vi "SMU.SetVoltage.vi"(8 "error in (no error)":errorcluster, 10 "Voltage, V":dbl, 11 "SMU.Keithley2600 in":refnum<class "SMU.Keithley2600.lvclass">) -> (0 "error out":errorcluster, 3 "SMU.Keithley2600 out":refnum<class "SMU.Keithley2600.lvclass">)   [LabVIEW 2017, in "SMU.Keithley2600.lvclass"]
uses:
  SMU.Keithley2600.lvclass
  <instrlib>/Keithley 2600 Series/Public/Configure/Source/Configure Source (Level).vi
  <instrlib>/Keithley 2600 Series/Keithley 2600 Series.lvlib
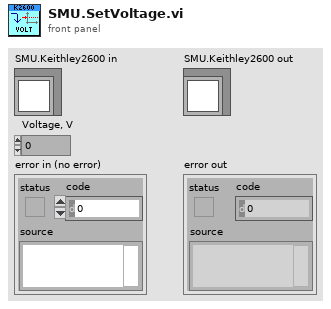
[diagram p1: front panel]
types:
  T1 = typedef "SMU.Keithley2600.lvclass/Resource--Cluster.ctl" = cluster{"VISA resource":refnum<visa-resource-name>, "Channel":i32}
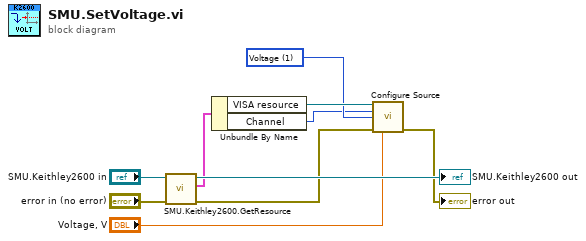
[diagram p0: block diagram]
diagram:
  w5 = 1 items=["Current", "Voltage"] ("Level Type (1: Voltage)")
  n1 = call "SMU.Keithley2600.GetResource.vi"("error in (no error)"="error in (no error)", "SMU.Keithley2600 in"="SMU.Keithley2600 in") -> ("error out"=w3:errorcluster, "Resource"=w7:T1, "SMU.Keithley2600 out"=→"SMU.Keithley2600 out":refnum<class "SMU.Keithley2600.lvclass">)  [unwired: 7 in]
  n2 = Unbundle By Name(w7) -> ("VISA resource"=w6:refnum<visa-resource-name>, "Channel"=w4:i32)
  n3 = call-poly <instrlib>:"Configure Source.vi"("VISA resource name"=w6, "Source Measure Unit Channel (0: Channel A)"=w4, "Level Type (1: Voltage)"=w5, "error in (no error)"=w3, "Voltage Level (0 V)"="Voltage, V") -> ("error out"=→"error out":errorcluster)  [unwired: 9 in, 1 out]
